vi "Video signl setup first call error.vi"   [LabVIEW 2013]
panel:
  # "Re-Entrant"
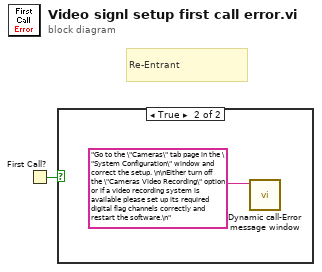
[diagram p0: block diagram]
diagram:
  # "Re-Entrant"
  n1 = First Call?() -> (First Call?: T/F=w1:bool)
  n2 = case shown="True" w1 {
    frame False {
    }
    frame True {
      n3 = call "Dynamic call-Error message window.vi"("Error Message"="Go to the \"Cameras\" tab page in the \"System Configuration\" window and correct the setup. \n\nEither turn off the \"Cameras Video Recording\" option or if a video recording system is available please set up its required digital flag channels correctly and restart the software.\n" ("format string")) -> ()  [unwired: 10 in, 1 out]
    }
  }
